vi "New.vi"(8 "error in (no error)":errorcluster, 10 "#bytes per timestamp":i32, 11 "Buffer Size (#timestamps)":i32) -> (0 "error out":errorcluster, 3 "Ring buffer DVR":refnum<data-value>)   [LabVIEW 2021, in "Ring Buffer Time Series Data.lvlib"]
uses:
  Ring Buffer Time Series Data.lvlib
  SubVIs/DVR data.ctl
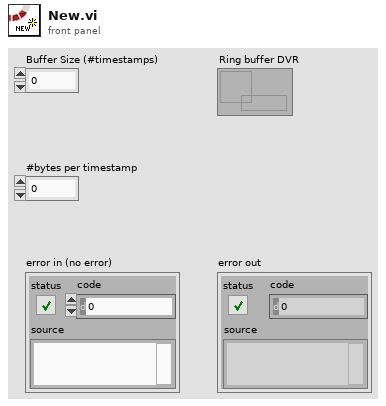
[diagram p1: front panel]
types:
  T1 = typedef "Ring Buffer Time Series Data.lvlib/DVR data.ctl" = cluster{"Timestamps":u64[], "Values":u8[], "#bytes per timestamp":i32, "Index":i32, "Size (#timestamps)":i32, "Full?":bool}
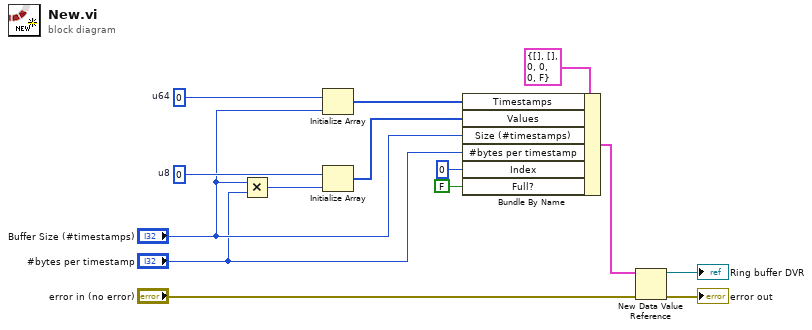
[diagram p0: block diagram]
diagram:
  w12 = u64 0  # u64
  w13 = u8 0  # u8
  n1 = Multiply(x="Buffer Size (#timestamps)", y="#bytes per timestamp") -> (x*y=w11:i32)
  n2 = Initialize Array(w12, "Buffer Size (#timestamps)") -> (w9:u64[])
  n3 = Initialize Array(w13, w11) -> (w8:u8[])
  n4 = Bundle By Name(cluster=T1 {"Timestamps"=[], "Values"=[], "#bytes per timestamp"=0, "Index"=0, "Size (#timestamps)"=0, "Full?"=FALSE} ("Cluster"), "Timestamps"=w9, "Values"=w8, "Size (#timestamps)"="Buffer Size (#timestamps)", "#bytes per timestamp"="#bytes per timestamp", "Index"=0 ("data size"), "Full?"=FALSE) -> (w5:T1)
  n5 = New Data Value Reference(data value=w5, error in="error in (no error)") -> (data value reference=→"Ring buffer DVR":refnum<data-value>, error out=→"error out":errorcluster)
